vi "PRODUCTOR AND CONSUMER.vi"() -> ()   [LabVIEW 2018]
panel:
  in  "error in (read msg)":errorcluster
  in  "VISA resource name out":refnum<visa-resource-name>
  in  "stop":bool
  in  "milliseconds to wait":u32
  out "msg answer":string
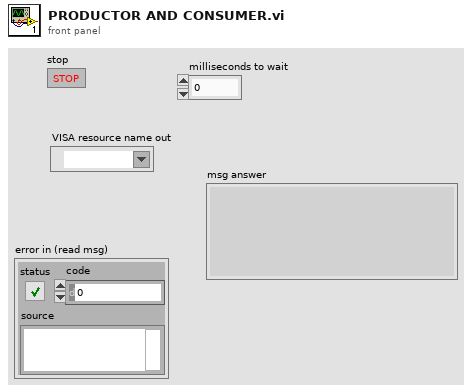
[diagram p1: front panel]
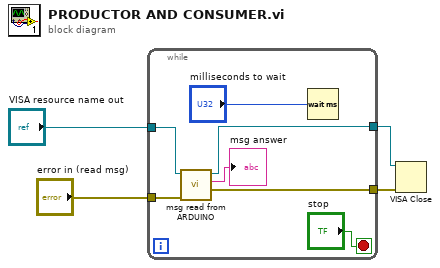
[diagram p0: block diagram]
diagram:
  n1 = while {
    tunnel: "VISA resource name out" -> [w11]
    tunnel: [w8] -> w4
    tunnel: [w7] -> w3
    tunnel: "error in (read msg)" -> [w5]
    stop <- "stop" stop-if-true
    n2 = call "msg read from ARDUINO.vi"("error in (read msg)"=w5, "VISA Refnum in"=w11) -> ("error out (read msg)"=w7:errorcluster, "msg answer"=→"msg answer":string, "VISA Refnum out"=w8:refnum<visa-resource-name>)  [unwired: 7 in]
    n3 = Wait (ms)(milliseconds to wait="milliseconds to wait") -> ()  [unwired: 1 out]
  }
  n4 = VISA Close(VISA resource name=w4, error in (no error)=w3) -> ()  [unwired: 1 out]
